vi "exercise3_paintsine.vi"() -> ()   [LabVIEW 2018]
panel:
  out "Output: Waveform Chart":dbl(graph)
  in  "dt":dbl
  out "Numeric":dbl
  in  "amplitud":dbl
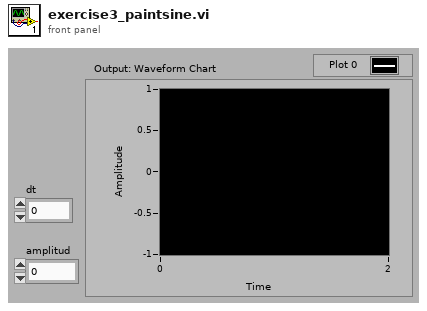
[diagram p1: front panel]
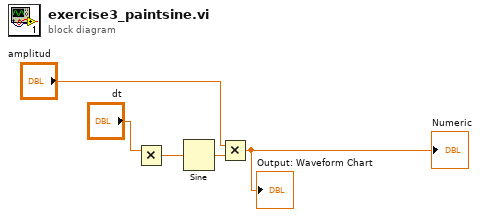
[diagram p0: block diagram]
diagram:
  n1 = Multiply(x="dt") -> (x*y=w1:dbl)  [unwired: 1 in]
  n2 = Sine(x=w1) -> (sin(x)=w3:dbl)
  n3 = Multiply(x="amplitud", y=w3) -> (x*y=→"Numeric" →"Output: Waveform Chart":dbl)
